vi "Sum scalar.vi"() -> ()   [LabVIEW 2015]
panel:
  in  "stop":bool
  in  "y":dbl
  in  "x":dbl
  out "SUM (MATLAB)":dbl
  out "SUM (formula node)":dbl
  out "SUM (Native)":dbl
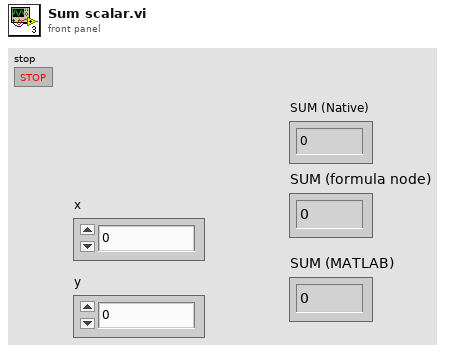
[diagram p1: front panel]
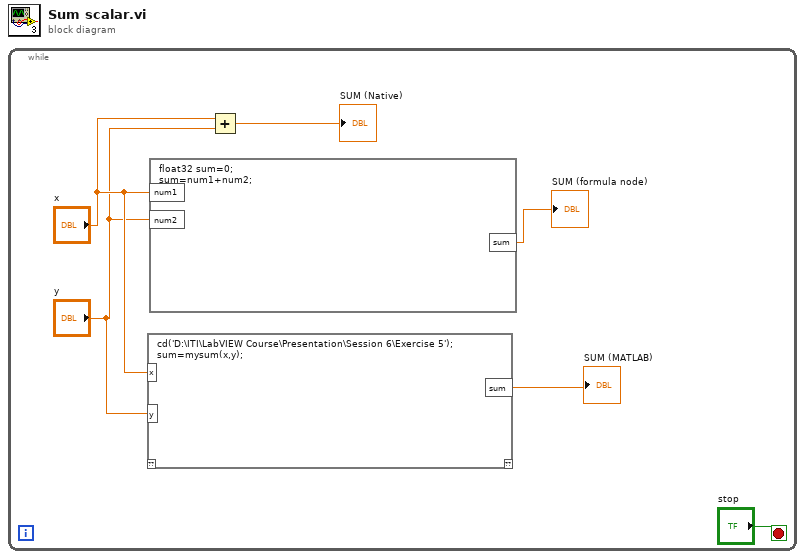
[diagram p0: block diagram]
diagram:
  n1 = while {
    stop <- "stop" stop-if-true
    n2 = script code="cd('D:\\ITI\\LabVIEW Course\\Presentation\\Session 6\\Exercise 5');\nsum=mysum(x,y);"("x"="x", "y"="y") -> ("sum"=→"SUM (MATLAB)":dbl)  [unwired: 1 in, 1 out]
    n3 = formula code="float32 sum=0;\nsum=num1+num2;"("num1"="x", "num2"="y") -> ("sum"=→"SUM (formula node)":sgl)
    n4 = Add(x="x", y="y") -> (x+y=→"SUM (Native)":dbl)
  }
